vi "SP Limit Test Inside.vi"(5 "x0":dbl format="%0.2f", 7 "dx":dbl=1.0 format="%0.2f", 8 "limit test config":T2={"pass region"=0, "include UL"=TRUE, "include LL"=TRUE} {"pass region" items=["inside limits", "outside limits"]}, 9 "lower":dbl[](array[numeric]) format="%0.2f", 10 "upper":dbl[](array[numeric]) format="%0.2f", 11 "signal":dbl[](array[numeric]) format="%0.2f") -> (0 "clearance":T1 {"min clearance" format="%.2f"; "clearance LL" format="%.2f"; "clearance UL" format="%.2f"}, 1 "failures":cluster{"x values":dbl[], "y values":dbl[]} {"y values" format="%.2f"; "x values" format="%.2f"}, 2 "test results":bool[](array[boolean]), 3 "Y":dbl[](array[numeric]) format="%0.2f")   [LabVIEW 2011]
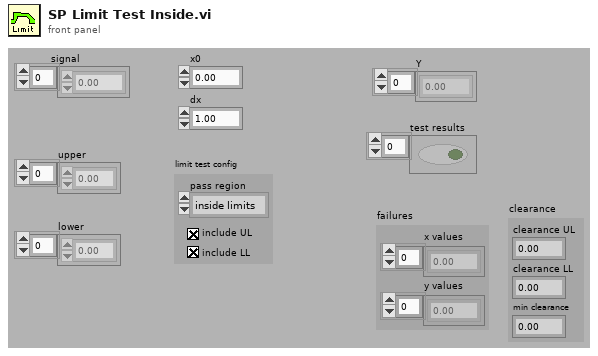
[diagram p1: front panel]
types:
  T1 = cluster{"clearance UL":dbl, "clearance LL":dbl, "min clearance":dbl}
  T2 = cluster{"pass region":i32, "include UL":bool, "include LL":bool}
  T3 = cluster{"clearanceUL":dbl, "clearanceUL":dbl, dbl}
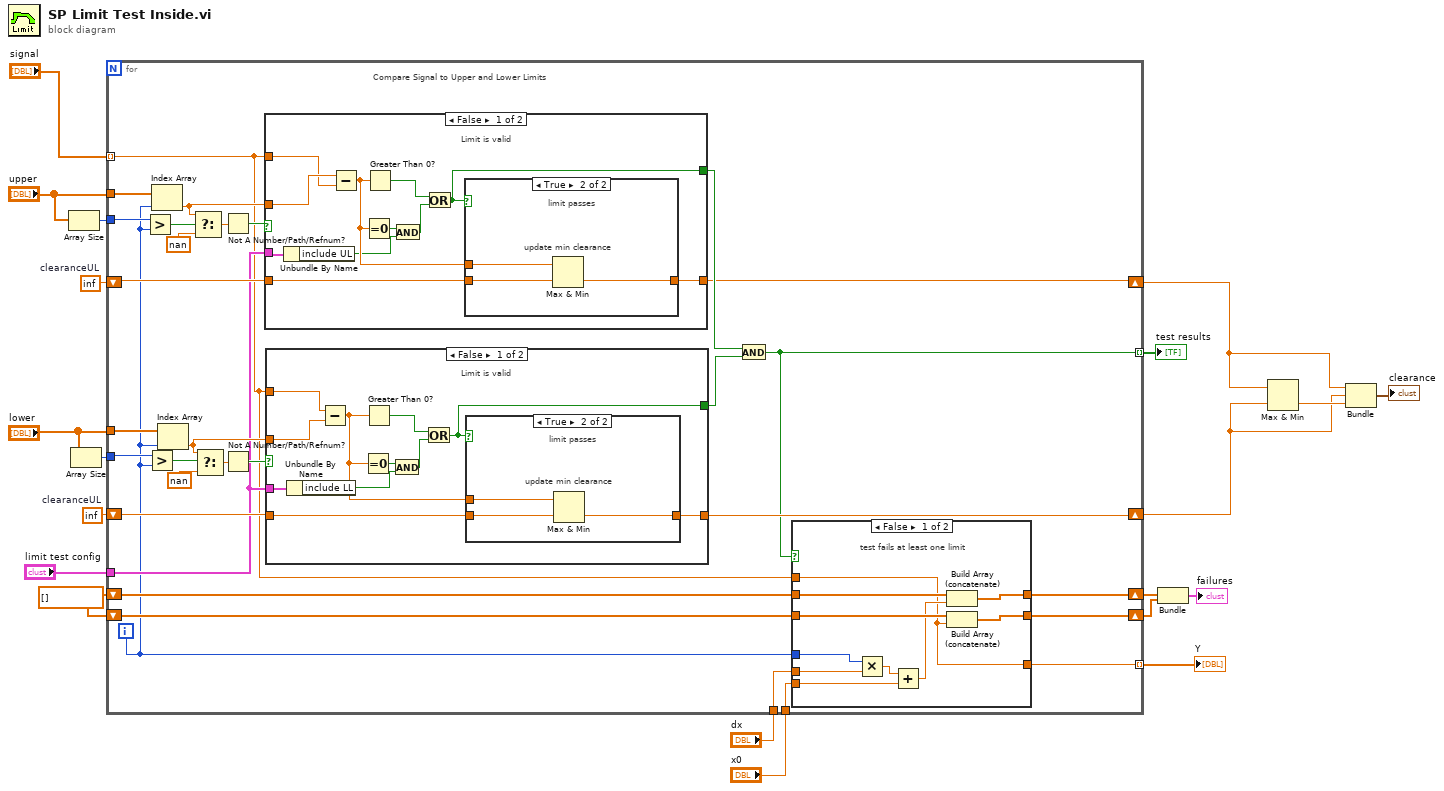
[diagram p0: block diagram]
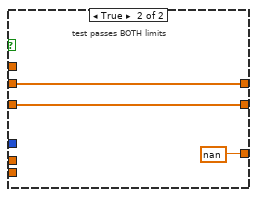
[diagram p2: hidden frame]
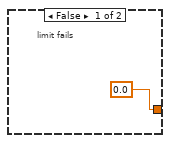
[diagram p3: hidden frame]
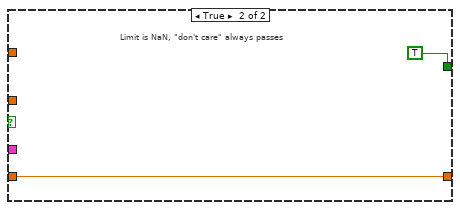
[diagram p4: hidden frame]
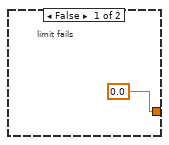
[diagram p5: hidden frame]
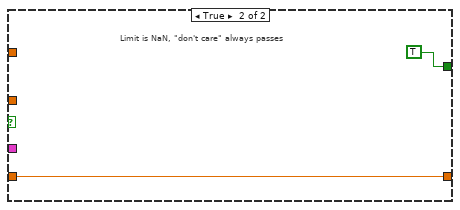
[diagram p6: hidden frame]
diagram:
  w15 = dbl[] [] ("x values")
  w16 = inf  # clearanceUL
  w18 = inf  # clearanceUL
  n1 = Array Size(array="upper") -> (size(s)=w20:i32)
  n2 = Array Size(array="lower") -> (size(s)=w19:i32)
  n3 = for {
    tunnel: "upper" -> [w45]
    tunnel: "signal" -> [w23] mode=indexing
    tunnel: "lower" -> [w44]
    tunnel: w20 -> [w51]
    tunnel: w19 -> [w47]
    tunnel: "limit test config" -> [w35]
    shift-right: [w29] -> w9
    shift-left: w18 -> [w40]
    shift-right: [w30] -> w8
    shift-left: w16 -> [w36]
    shift-right: [w27] -> w14
    shift-left: w15 -> [w32]
    shift-right: [w26] -> w13
    shift-left: w15 -> [w31]
    tunnel: [w25] -> w11 mode=indexing
    tunnel: [w24] -> w6 mode=indexing
    tunnel: "dx" -> [w22]
    tunnel: "x0" -> [w21]
    i -> [w28]
    # "Compare Signal to Upper and Lower Limits"
    n4 = Greater?(x=w51, y=w28) -> (0:w50:bool)
    n5 = Greater?(x=w47, y=w28) -> (0:w46:bool)
    n6 = Index Array(array=w45, index=w28) -> (element=w41:dbl)
    n7 = Index Array(array=w44, index=w28) -> (element=w37:dbl)
    n8 = Select(t=w41, s=w50, f=nan ("t")) -> (s? t:f=w43:dbl)
    n9 = Select(t=w37, s=w46, f=nan ("t")) -> (s? t:f=w39:dbl)
    n10 = Not A Number/Path/Refnum?(number/path/refnum=w43) -> (NaN/Path/Refnum?=w42:bool)
    n11 = Not A Number/Path/Refnum?(number/path/refnum=w39) -> (NaN/Path/Refnum?=w38:bool)
    n12 = case shown="False" w42 {
      tunnel: w41 -> [w92 _]
      tunnel: w23 -> [w91 _]
      tunnel: w35 -> [w83 _]
      tunnel: w40 -> [w87 w98]
      tunnel: [w85 w98] -> w29
      tunnel: [w82 TRUE] -> w34
      frame False {
        # "Limit is valid"
        n13 = Unbundle By Name(w83) -> ("include UL"=w84:bool)
        n14 = Subtract(x=w92, y=w91) -> (x-y=w86:dbl)
        n15 = Equal To 0?(x=w86) -> (x = 0?=w90:bool)
        n16 = Greater Than 0?(x=w86) -> (x > 0?=w89:bool)
        n17 = And(x=w90, y=w84) -> (x .and. y?=w88:bool)
        n18 = Or(x=w89, y=w88) -> (x .or. y?=w82:bool)
        n19 = case shown="True" w82 {
          tunnel: w87 -> [_ w95]
          tunnel: [0.0 w94] -> w85
          tunnel: w86 -> [_ w96]
          frame False {
            # "limit fails"
          }
          frame True {
            # "update min clearance"
            # "limit passes"
            n20 = Max & Min(x=w96, y=w95) -> (min(x,y)=w94:dbl)  [unwired: 1 out]
          }
        }
      }
      frame True {
        # "Limit is NaN, \"don't care\" always passes"
      }
    }
    n21 = case shown="False" w38 {
      tunnel: w37 -> [w75 _]
      tunnel: w23 -> [w74 _]
      tunnel: w36 -> [w70 w81]
      tunnel: [w68 w81] -> w30
      tunnel: w35 -> [w67 _]
      tunnel: [w65 TRUE] -> w33
      frame False {
        # "Limit is valid"
        n22 = Unbundle By Name(w67) -> ("include LL"=w66:bool)
        n23 = Subtract(x=w74, y=w75) -> (x-y=w69:dbl)
        n24 = Equal To 0?(x=w69) -> (x = 0?=w73:bool)
        n25 = Greater Than 0?(x=w69) -> (x > 0?=w72:bool)
        n26 = And(x=w73, y=w66) -> (x .and. y?=w71:bool)
        n27 = Or(x=w72, y=w71) -> (x .or. y?=w65:bool)
        n28 = case shown="True" w65 {
          tunnel: w70 -> [_ w78]
          tunnel: [0.0 w77] -> w68
          tunnel: w69 -> [_ w79]
          frame False {
            # "limit fails"
          }
          frame True {
            # "update min clearance"
            # "limit passes"
            n29 = Max & Min(x=w79, y=w78) -> (min(x,y)=w77:dbl)  [unwired: 1 out]
          }
        }
      }
      frame True {
        # "Limit is NaN, \"don't care\" always passes"
      }
    }
    n30 = And(x=w34, y=w33) -> (x .and. y?=w25:bool)
    n31 = case shown="False" w25 {
      tunnel: w32 -> [w61 w64]
      tunnel: w31 -> [w60 w63]
      tunnel: w28 -> [w58 _]
      tunnel: w23 -> [w54 _]
      tunnel: [w56 w64] -> w27
      tunnel: [w55 w63] -> w26
      tunnel: [w54 nan] -> w24
      tunnel: w22 -> [w53 _]
      tunnel: w21 -> [w52 _]
      frame False {
        # "test fails at least one limit"
        n32 = Multiply(x=w58, y=w53) -> (x*y=w59:dbl)
        n33 = Add(x=w59, y=w52) -> (x+y=w57:dbl)
        n34 = Build Array (concatenate)(w61, w57) -> (w56:dbl[])
        n35 = Build Array (concatenate)(w60, w54) -> (w55:dbl[])
      }
      frame True {
        # "test passes BOTH limits"
      }
    }
  }
  "test results" <- w11
  "Y" <- w6
  n36 = Bundle("x values"=w14, "x values"=w13) -> (→"failures":cluster{"x values":dbl[], "x values":dbl[]})  [unwired: 1 out]
  n37 = Max & Min(x=w9, y=w8) -> (min(x,y)=w10:dbl)  [unwired: 1 out]
  n38 = Bundle("clearanceUL"=w9, "clearanceUL"=w8, w10) -> (→"clearance":T3)  [unwired: 1 out]
